vi "CRYGraph Text Window.vi"() -> ()   [LabVIEW 2013]
uses:
  Control/CRYFlag Cluster.ctl
  SubVI/CRYData View Global.vi
  SubVI/CRYMain Sub Window Global.vi
  CRYCurveLibrary/Global/CRYCurve Library Global.vi
panel:
  out "Event Name":string
  out "PropertyTab":string
  in  "OpenProperty":bool
  out "Test":string
  in  "Cursor":string[][](table)
  out "Cursor Ref":refnum<vi>
  out "Queue Name":string
  in  "StateOut":bool
  in  "CursorShow":bool
  out "Graph Number":i32
  in  "LegendShow":bool
  out "Graph Ref":refnum<vi>
  in  "Legend":i32(listbox) caption="Multicolumn Listbox"
  out "Legend Ref":refnum<vi>
  in  "GraphType":string
  out "Title Name":string
  in  "stop":bool
  in  "GText":string
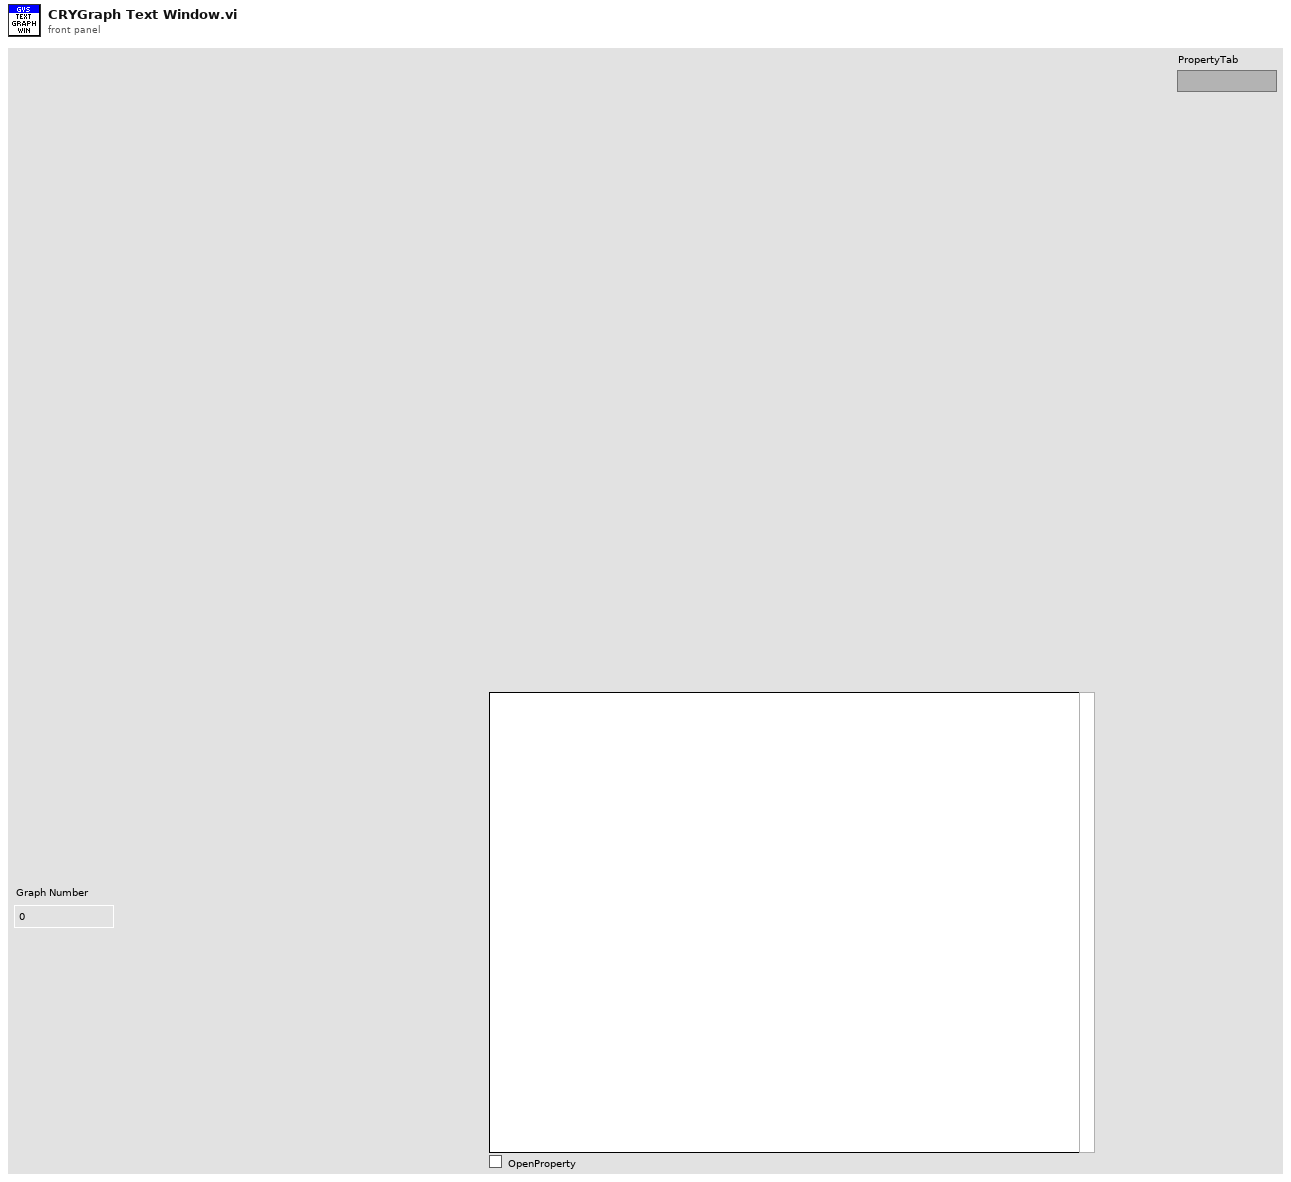
[diagram p1: front panel]
types:
  T1 = typedef "CRYGraph Event.ctl" = cluster{"EvenName":string, "TitleName":string, "GraphName":string, "GraphType":string, "Data":variant, "Queue Name":string, "DataView Number":i32}
  T2 = typedef "CRYFlag Cluster.ctl" = cluster{"LegendShow":bool, "CellClick":bool, "Total Number":bool, "ScaleFitX":bool, "ScaleFitY":bool, "MapModeX":u8, "MapModeY":u8, "CursorShow":bool, "MagnitudeShow":bool, "PreviewShow":bool, "CursorEnabled":bool, "IntensityShow":bool, "PaletteShow":bool, "PhaseShow":bool, "XYShow":bool, "FrequencyShow":bool, "LegendVScrollShow":bool, "FrequencyVScrollShow":bool}
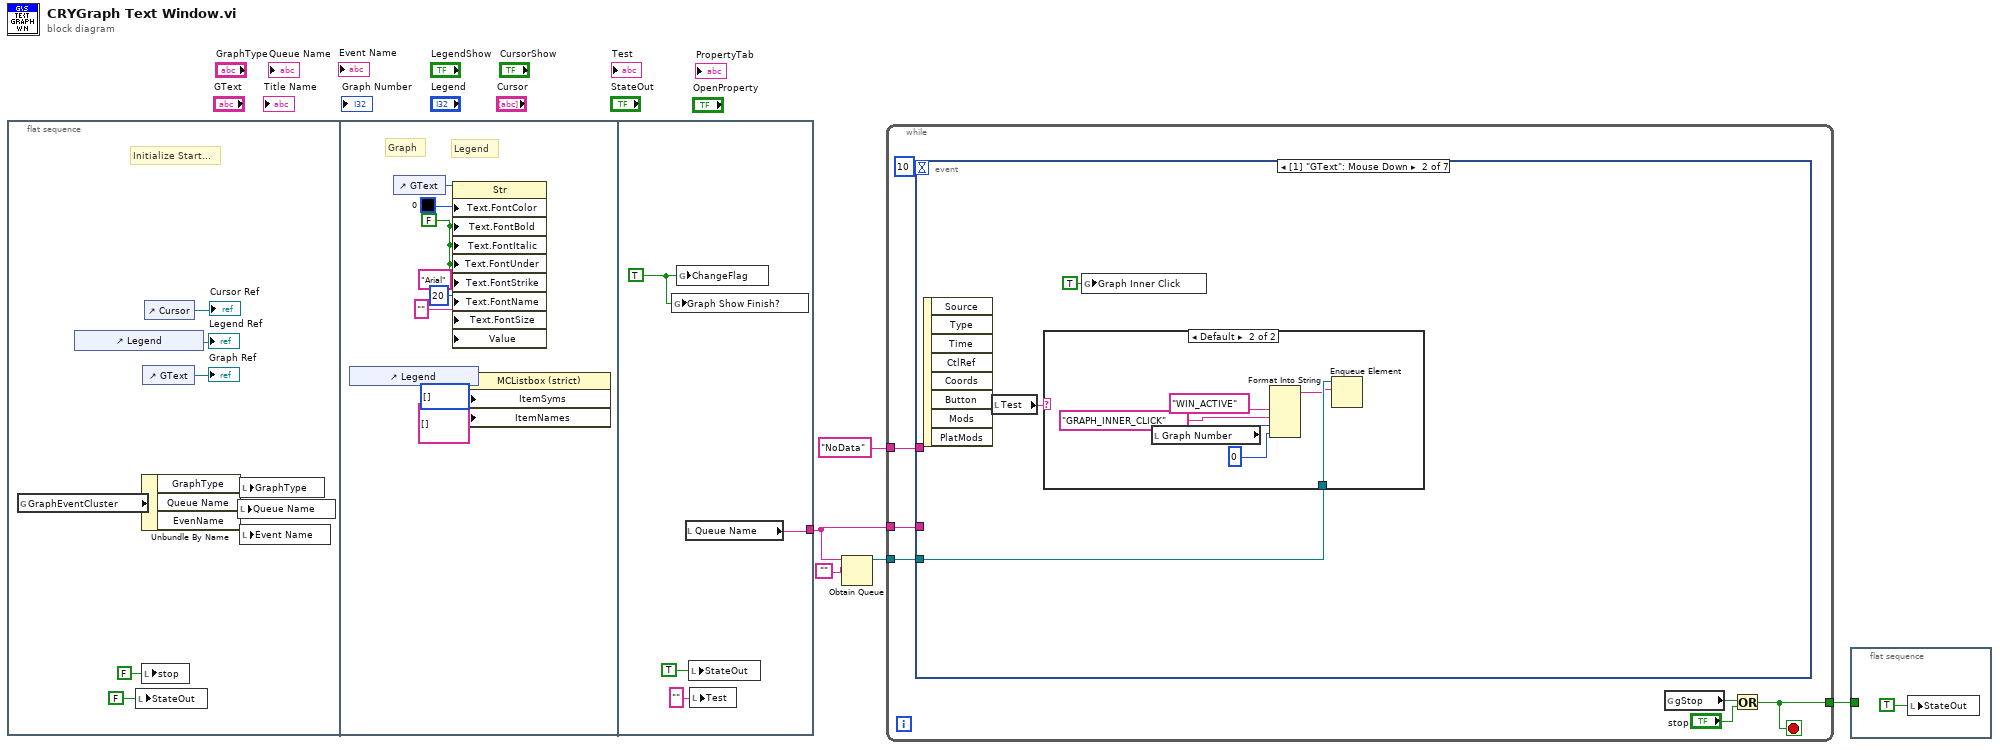
[diagram p0: block diagram]
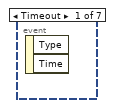
[diagram p2: hidden frame]
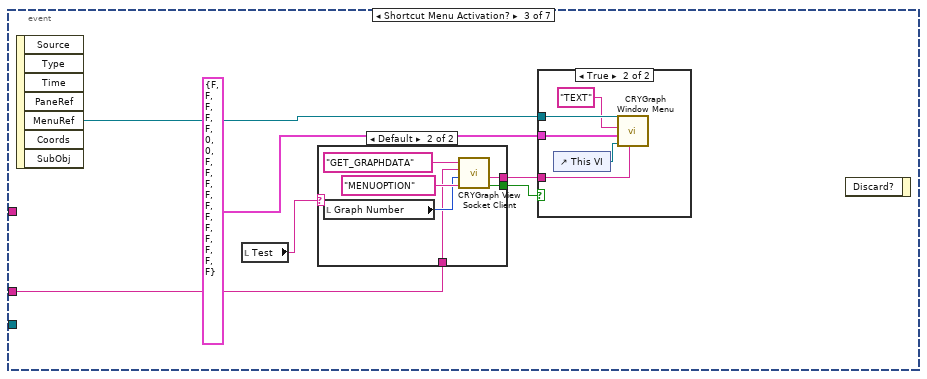
[diagram p4: hidden frame]
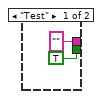
[diagram p5: hidden frame]
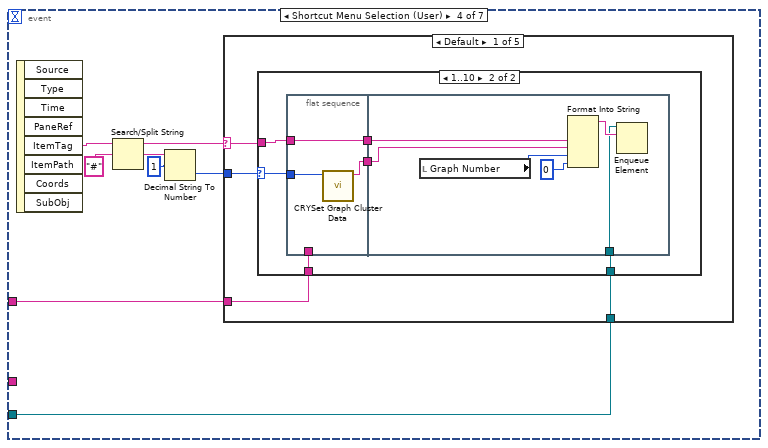
[diagram p7: hidden frame]
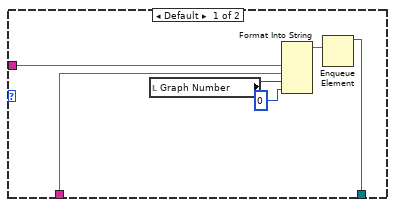
[diagram p8: hidden frame]
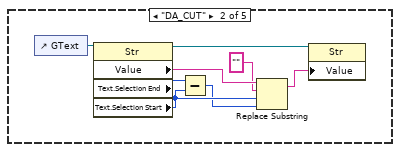
[diagram p9: hidden frame]
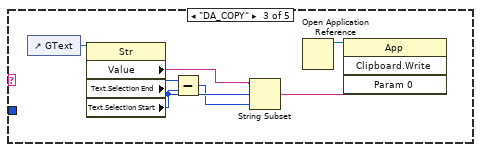
[diagram p10: hidden frame]
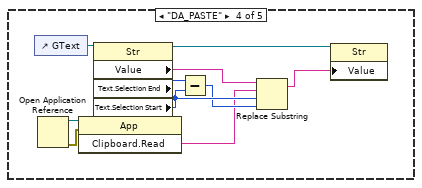
[diagram p11: hidden frame]
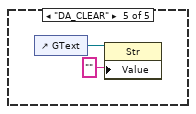
[diagram p12: hidden frame]
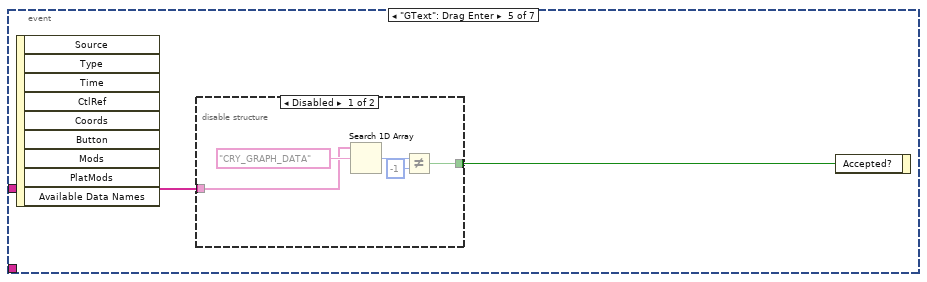
[diagram p13: hidden frame]
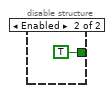
[diagram p14: hidden frame]
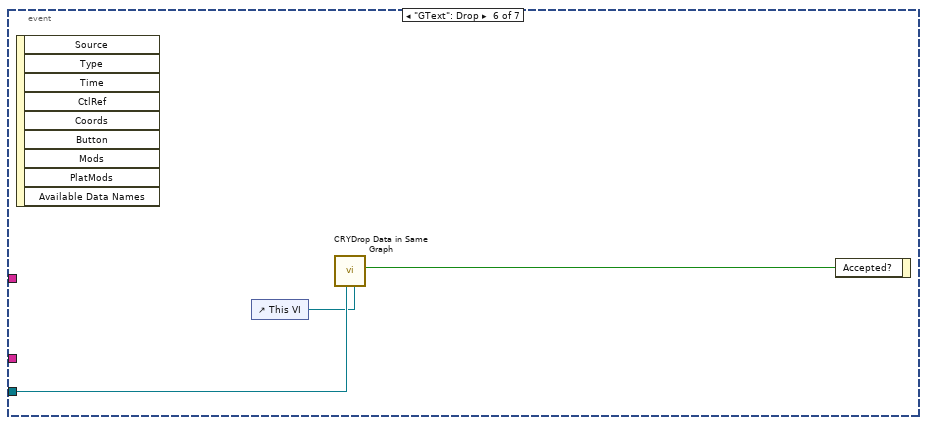
[diagram p15: hidden frame]
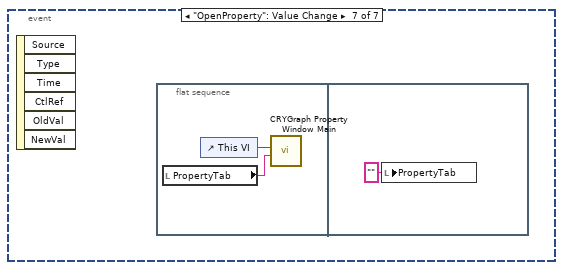
[diagram p16: hidden frame]
diagram:
  n1 = flat-sequence {
    tunnel: [w24] -> w2
    frame #0 {
      # "Initialize Start..."
      n2 = global read "CRYData View Global.vi" "GraphEventCluster"() -> (w7:T1)
      n3 = control-ref of="Legend"() -> (→"Legend Ref":refnum<vi>)
      n4 = local write "StateOut"(FALSE ("StateOut")) -> ()
      n5 = Unbundle By Name(w7) -> ("GraphType"=w8:string, "Queue Name"=w9:string, "EvenName"=w6:string)
      n6 = local write "stop"(FALSE ("stop")) -> ()
      n7 = control-ref of="GText"() -> (→"Graph Ref":refnum<vi>)
      n8 = control-ref of="Cursor"() -> (→"Cursor Ref":refnum<vi>)
      n9 = local write "Queue Name"(w9) -> ()
      n10 = local write "GraphType"(w8) -> ()
      n11 = local write "Event Name"(w6) -> ()
    }
    frame #1 {
      w21 = FALSE ("Text.Font:Bold")
      # "Legend"
      # "Graph"
      n12 = control-ref of="Legend"() -> (w18:refnum<vi>)
      n13 = control-ref of="GText"() -> (w19:refnum<vi>)
      n14 = property class="Str"(reference=w19, "Text.FontColor"=u32 0, "Text.FontBold"=w21, "Text.FontItalic"=w21, "Text.FontUnder"=w21, "Text.FontStrike"=w21, "Text.FontName"="Arial" ("Text.Font:Name"), "Text.FontSize"=u32 20 ("Text.Font:Size"), "Value"="") -> ()  [unwired: 1 in, 2 out]
      n15 = property on="Property Node" class="MCListbox (strict)"(reference=w18, "ItemSyms"=i32[] [] ("Item Symbols"), "ItemNames"=string[][] [] ("Item Names")) -> ()  [unwired: 1 in, 2 out]
    }
    frame #2 {
      w27 = TRUE ("ChangeFlag")
      n16 = global write "CRYData View Global.vi" "Graph Show Finish?"(w27) -> ()
      n17 = global write "CRYData View Global.vi" "ChangeFlag"(w27) -> ()
      n18 = local read "Queue Name"() -> (w24:string)
      n19 = local write "StateOut"(TRUE ("StateOut")) -> ()
      n20 = local write "Test"("" ("Test")) -> ()
    }
  }
  n21 = Obtain Queue(name (unnamed)=w2, element data type="") -> (queue out=w4:refnum<queue>)  [unwired: 3 in, 2 out]
  n22 = while {
    tunnel: w4 -> [w34]
    tunnel: "NoData" ("input 2") -> [w33]
    tunnel: w2 -> [w31]
    tunnel: [w28] -> w1
    stop <- w28 stop-if-true
    n23 = event shown="[1] \"GText\": Mouse Down" {
      selector: _ -> [_ _ _ _ _ _ _]
      dyn-events: _ -> [_ _ _ _ _ _ _]
      timeout: 10 -> [_ _ _ _ _ _ _]
      tunnel: w34 -> [_ w37 _ w65 _ w132 _]
      tunnel: w33 -> [_ _ _ w64 _ _ _]
      tunnel: w31 -> [_ _ w45 _ _ _ _]
      event Timeout {
        n24 = event-data() -> ()  [unwired: 3 out]
      }
      event "GText": Mouse Down {
        n25 = event-data() -> ()  [unwired: 9 out]
        n26 = local read "Test"() -> (w36:string)
        n27 = case shown="Default" w36 {
          tunnel: w37 -> [_ w43]
          frame "Test" {
          }
          frame Default {
            n28 = local read "Graph Number"() -> (w42:i32)
            n29 = Format Into String("WIN_ACTIVE" ("input 1"), "GRAPH_INNER_CLICK" ("input 1"), w42, 0 ("input 3")) -> (resulting string=w40:string)  [unwired: 3 in, 1 out]
            n30 = Enqueue Element(queue=w43, element=w40) -> ()  [unwired: 1 in, 4 out]
          }
        }
        n31 = global write "CRYCurve Library Global.vi" "Graph Inner Click"(TRUE ("Graph Inner Click")) -> ()
      }
      event Shortcut Menu Activation? {
        n32 = event-data() -> ("MenuRef"=w47:refnum<k9>)  [unwired: 7 out]
        n33 = local read "Test"() -> (w44:string)
        n34 = case shown="Default" w44 {
          tunnel: ["" ("sData Out") w55] -> w49
          tunnel: [TRUE ("bResult Out") w54] -> w48
          tunnel: w45 -> [_ w52]
          frame "Test" {
          }
          frame Default {
            n35 = local read "Graph Number"() -> (w53:i32)
            n36 = call "CRYGraph View Socket Client.vi"("sOption"="MENUOPTION", "nData"=w53, "sData"=w52, "sAction"="GET_GRAPHDATA") -> ("bResult Out"=w54:bool, "sData Out"=w55:string)  [unwired: 4 in, 2 out]
          }
        }
        n37 = case shown="True" w48 {
          tunnel: w47 -> [_ w62]
          tunnel: T2 {"LegendShow"=FALSE, "CellClick"=FALSE, "Total Number"=FALSE, "ScaleFitX"=FALSE, "ScaleFitY"=FALSE, "MapModeX"=0, "MapModeY"=0, "CursorShow"=FALSE, "MagnitudeShow"=FALSE, "PreviewShow"=FALSE, "CursorEnabled"=FALSE, "IntensityShow"=FALSE, "PaletteShow"=FALSE, "PhaseShow"=FALSE, "XYShow"=FALSE, "FrequencyShow"=FALSE, "LegendVScrollShow"=FALSE, "FrequencyVScrollShow"=FALSE} ("Flag Cluster") -> [_ w60]
          tunnel: w49 -> [_ w59]
          frame False {
          }
          frame True {
            n38 = control-ref of="This VI"() -> (w58:refnum<vi>)
            n39 = call "CRYGraph Window Menu.vi"("MenuOption"=w59, "pGraph VI"=w58, "Flag Cluster"=w60, "Type"="TEXT", "Runtime Menu Ref In"=w62) -> ()  [unwired: 7 out]
          }
        }
        n40 = event-data() -> ()  [unwired: 1 in, 2 out]
      }
      event Shortcut Menu Selection (User) {
        n41 = event-data() -> ("ItemTag"=w66:string)  [unwired: 8 out]
        n42 = Search/Split String(string=w66, search string/char (-)="#") -> (substring before match=w63:string, match + rest of string=w68:string)  [unwired: 2 out]
        n43 = Decimal String To Number(string=w68, offset=1) -> (number=w70:i32)  [unwired: 2 out]
        n44 = case shown="Default" w63 {
          selector: w63 -> [w71 _ _ _ _]
          tunnel: w70 -> [w74 _ _ _ _]
          tunnel: w65 -> [w73 _ _ _ _]
          tunnel: w64 -> [w72 _ _ _ _]
          frame Default {
            n45 = case shown="1..10" w74 {
              selector: w74 -> [_ w83]
              tunnel: w71 -> [w77 w86]
              tunnel: w73 -> [w78 w85]
              tunnel: w72 -> [w75 w82]
              frame Default {
                n46 = local read "Graph Number"() -> (w76:i32)
                n47 = Format Into String(w77, w75, w76, 0 ("input 3")) -> (resulting string=w79:string)  [unwired: 3 in, 1 out]
                n48 = Enqueue Element(queue=w78, element=w79) -> ()  [unwired: 1 in, 4 out]
              }
              frame 1..10 {
                n49 = flat-sequence {
                  tunnel: w86 -> [w89]
                  tunnel: [w89] -> w84
                  tunnel: w83 -> [w88]
                  tunnel: w82 -> [_]
                  tunnel: [w87] -> w81
                  tunnel: w85 -> [w93]
                  tunnel: w84 -> [w92]
                  tunnel: w81 -> [w90]
                  frame #0 {
                    n50 = call "CRYSet Graph Cluster Data.vi"("Graph Number"=w88) -> ("DataType"=w87:string)  [unwired: 2 in, 8 out]
                  }
                  frame #1 {
                    n51 = local read "Graph Number"() -> (w91:i32)
                    n52 = Format Into String(w92, w90, w91, 0 ("input 3")) -> (resulting string=w95:string)  [unwired: 3 in, 1 out]
                    n53 = Enqueue Element(queue=w93, element=w95) -> ()  [unwired: 1 in, 4 out]
                  }
                }
              }
            }
          }
          frame "DA_CUT" {
            n54 = control-ref of="GText"() -> (w103:refnum<vi>)
            n55 = property class="Str"(reference=w103) -> (reference out=w97:refnum<vi>, "Value"=w101:string, "Text.Selection End"=w102:u32, "Text.Selection Start"=w99:u32)  [unwired: 1 in, 1 out]
            n56 = Subtract(x=w102, y=w99) -> (x-y=w98:u32)
            n57 = Replace Substring(2:w98, 3:w99, 4:"" ("substring (\"\")"), 5:w101) -> (1:w96:string)  [unwired: 1 out]
            n58 = property class="Str"(reference=w97, "Value"=w96) -> ()  [unwired: 1 in, 2 out]
          }
          frame "DA_COPY" {
            n59 = control-ref of="GText"() -> (w110:refnum<vi>)
            n60 = property class="Str"(reference=w110) -> ("Value"=w106:string, "Text.Selection End"=w109:u32, "Text.Selection Start"=w108:u32)  [unwired: 1 in, 2 out]
            n61 = Subtract(x=w109, y=w108) -> (x-y=w107:u32)
            n62 = String Subset(string=w106, offset (0)=w108, length (rest)=w107) -> (substring=w104:string)
            n63 = Open Application Reference() -> (3:w105:refnum<vi>)  [unwired: 4 in, 1 out]
            n64 = invoke class="App" method="Clipboard.Write"(reference=w105, "Param 0"=w104) -> ()  [unwired: 2 in, 4 out]
          }
          frame "DA_PASTE" {
            n65 = control-ref of="GText"() -> (w120:refnum<vi>)
            n66 = Open Application Reference() -> (0:w114:errorcluster, 3:w115:refnum<vi>)  [unwired: 4 in]
            n67 = invoke class="App" method="Clipboard.Read"(reference=w115, error in=w114) -> ("Read Clipbrd"=w113:string)  [unwired: 1 in, 2 out]
            n68 = property class="Str"(reference=w120) -> (reference out=w112:refnum<vi>, "Value"=w116:string, "Text.Selection End"=w119:u32, "Text.Selection Start"=w118:u32)  [unwired: 1 in, 1 out]
            n69 = Subtract(x=w119, y=w118) -> (x-y=w117:u32)
            n70 = Replace Substring(2:w117, 3:w118, 4:w113, 5:w116) -> (1:w111:string)  [unwired: 1 out]
            n71 = property class="Str"(reference=w112, "Value"=w111) -> ()  [unwired: 1 in, 2 out]
          }
          frame "DA_CLEAR" {
            n72 = control-ref of="GText"() -> (w121:refnum<vi>)
            n73 = property class="Str"(reference=w121, "Value"="") -> ()  [unwired: 1 in, 2 out]
          }
        }
      }
      event "GText": Drag Enter {
        n74 = event-data() -> ("Available Data Names"=w124:string[])  [unwired: 9 out]
        n75 = disable-structure shown="Disabled" {
          disable-tunnel: w124 -> [w126 _]
          disable-tunnel: [w125 TRUE] -> w123
          frame Disabled {
            n76 = Search 1D Array(1D array=w126, element="CRY_GRAPH_DATA") -> (index of element=w127:i32)  [unwired: 1 out]
            n77 = Not Equal?(x=w127, y=-1) -> (x != y?=w125:bool)
          }
          frame Enabled {
          }
        }
        n78 = event-data("Accepted?"=w123) -> ()  [unwired: 1 in, 1 out]
      }
      event "GText": Drop {
        n79 = event-data() -> ()  [unwired: 10 out]
        n80 = control-ref of="This VI"() -> (w131:refnum<vi>)
        n81 = call "CRYDrop Data in Same Graph.vi"("pGraph VI"=w131, "Queue"=w132) -> ("Accepted?"=w133:bool)  [unwired: 5 in, 4 out]
        n82 = event-data("Accepted?"=w133) -> ()  [unwired: 1 in, 1 out]
      }
      event "OpenProperty": Value Change {
        n83 = event-data() -> ()  [unwired: 7 out]
        n84 = flat-sequence {
          frame #0 {
            n85 = local read "PropertyTab"() -> (w134:string)
            n86 = control-ref of="This VI"() -> (w135:refnum<vi>)
            n87 = call "CRYGraph Property Window Main.vi"("TabName"=w134, "pGraph VI In"=w135) -> ()  [unwired: 1 in, 9 out]
          }
          frame #1 {
            n88 = local write "PropertyTab"("" ("PropertyTab")) -> ()
          }
        }
      }
    }
    n89 = global read "CRYMain Sub Window Global.vi" "gStop"() -> (w30:bool)
    n90 = Or(x=w30, y="stop") -> (x .or. y?=w28:bool)
  }
  n91 = flat-sequence {
    tunnel: w1 -> [_]
    frame #0 {
      n92 = local write "StateOut"(TRUE ("StateOut")) -> ()
    }
  }
